vi "Process.vi"(8 "error in (no error)":errorcluster, 10 "Pound in":refnum<class "Pound.lvclass">, 11 "Qbus in":refnum<class "Qbus.lvclass">) -> (0 "error out":errorcluster)   [LabVIEW 2017, in "CmsTestPanel.lvlib"]
uses:
  <vilib>/addons/InsightCM/Devices/Shared/Cms/CmsTestPanel/CmsTestPanel.lvlib
  <vilib>/addons/Qbus/Qbus.lvclass
  <vilib>/NI/Software Watchdog/Pound/Pound.lvclass
  <vilib>/addons/InsightCM/Devices/Shared/Cms/CmsTestPanel/controls/Configuration.ctl
  <vilib>/addons/InsightCM/Devices/Shared/Common/TestPanel/controls/Configuration.ctl
  <vilib>/addons/InsightCM/Devices/Shared/Common/TestPanel/controls/State.ctl
  <vilib>/addons/InsightCM/MessageBus/Base/controls/IRoutingSource.ctl
  <vilib>/addons/TraceLogger/TraceLogger.lvlib
  <vilib>/NI/Software Watchdog/Watchdog/Watchdog.lvclass
  <vilib>/addons/InsightCM/Devices/Shared/Common/DataFlow/DataFlow.lvlib
  <vilib>/addons/InsightCM/Utilities/GlobalConfiguration/GlobalConfiguration.lvlib
  <vilib>/addons/InsightCM/Devices/Shared/Common/ServerComm/ServerComm.lvlib
  <vilib>/addons/InsightCM/Devices/Shared/Common/TestPanel/TestPanel.lvlib
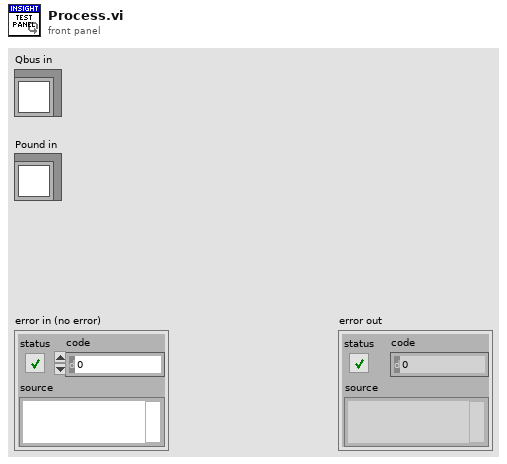
[diagram p1: front panel]
types:
  T1 = typedef "CmsTestPanel.lvlib/Configuration.ctl" = cluster{"Common":T2, "ChanNameMap":variant}
  T2 = typedef "TestPanel.lvlib/Configuration.ctl" = cluster{"State":T3, "Waveform Channel":string, "DataGroup":string, "Number of Samples":i32, "Waveform Length (sec)":dbl, "Timeout":dbl, "History":variant, "LastRequest":timestamp, "BufferSize":i32, "OpState":variant, "IRoutingSource":T4}
  T3 = typedef "TestPanel.lvlib/State.ctl" = enum16{"Off", "On", "PendingValues", "PendingDataSet"}
  T4 = typedef "IRoutingSource.ctl" = cluster{"CorrelationId":string, "ReplyTo":string}
  T5 = typedef "DataFlow.lvlib/Data.ctl" = cluster{"DataGroup":string, "Waveforms":T6, "Map":T7, "Type":T8}
  T6 = typedef "wfmSGL_DVR.ctl" = refnum<data-value>
  T7 = typedef "PointValueMap.lvlib/PointMap.ctl" = refnum<data-value>
  T8 = typedef "DataFlow.lvlib/Type.ctl" = enum16{"High Rate", "Low Rate", "Burst Mode"}
  T9 = typedef "Message.ctl" = cluster{"Header":T10, "Body":u8[]}
  T10 = typedef "MessageHeader.ctl" = cluster{"MessageName":string, "Timestamp":i64, "CorrelationId":string, "ContentType":string, "RoutingKey":string, "Properties":T11[]}
  T11 = typedef "KeyValuePair.ctl" = cluster{"Key":string, "Value":string}
  T12 = typedef "DeviceTestPanelGetTimeSeriesRequestBody.ctl" = cluster{"DataGroup":string, "TrendPointIds":string[]}
  T13 = typedef "DeviceTestPanelGetDataSetForChannelRequestBody.ctl" = cluster{"DataGroup":string, "ChannelName":string, "Properties":T11[]}
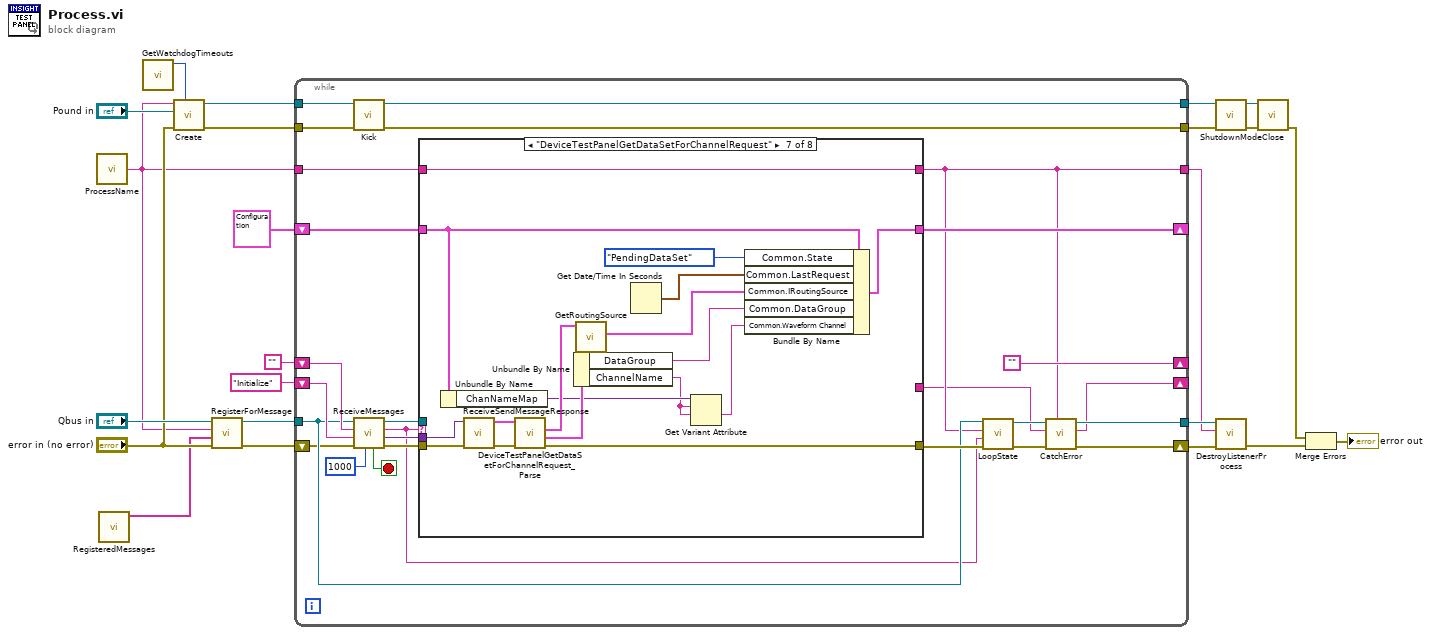
[diagram p0: block diagram]
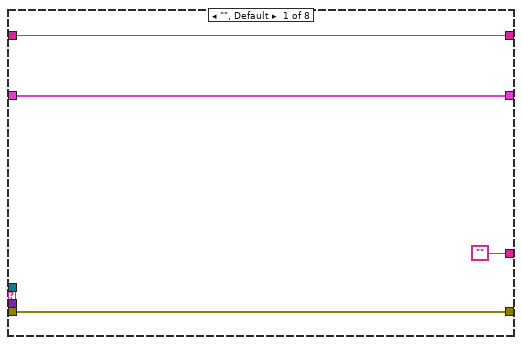
[diagram p2: hidden frame]
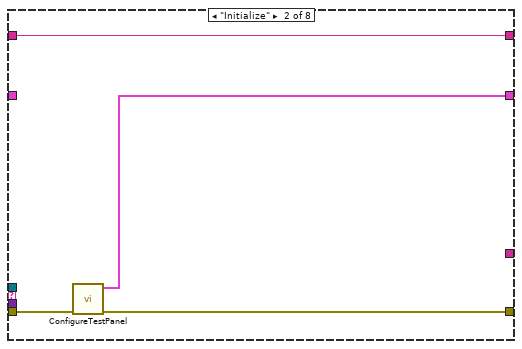
[diagram p3: hidden frame]
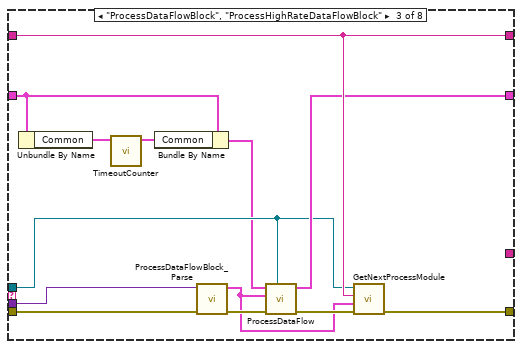
[diagram p4: hidden frame]
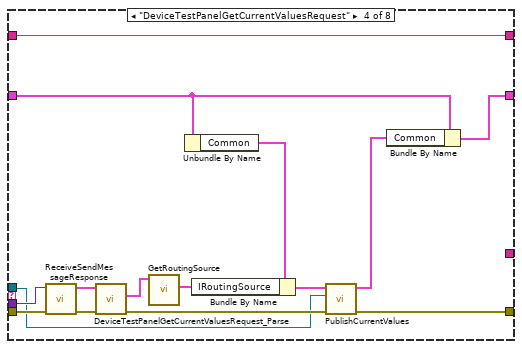
[diagram p5: hidden frame]
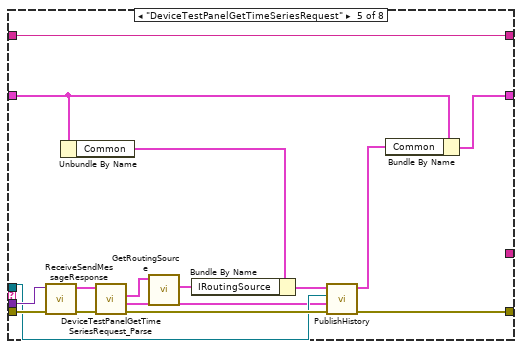
[diagram p6: hidden frame]
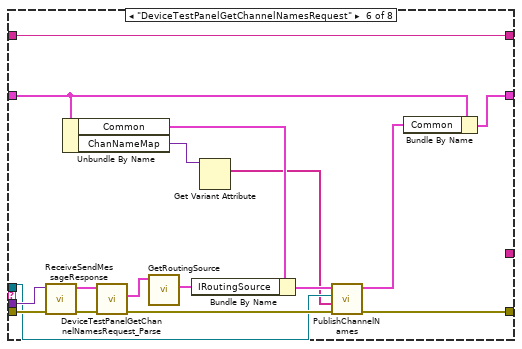
[diagram p7: hidden frame]
diagram:
  n1 = call <vilib>:"ProcessName.vi"() -> ("process name"=w3:string)  [unwired: 5 in]
  n2 = call <vilib>:"RegisteredMessages.vi"() -> ("registered messages"=w1:string[])  [unwired: 11 in]
  n3 = call <vilib>:"GetWatchdogTimeouts.vi"() -> ("software timeout"=w2:u32)  [unwired: 10 in, 1 out]
  n4 = call <vilib>:"Create.vi"("Execution Timeout (ms)"=w2, "error in (no error)"="error in (no error)", "Pound"="Pound in", "Name"=w3) -> ("error out"=w12:errorcluster, "Watchdog"=w17:refnum<data-value>)  [unwired: 6 in]
  n5 = call <vilib>:"RegisterForMessage.vi"("error in (no error)"="error in (no error)", "message names"=w1, "process name"=w3, "Qbus in"="Qbus in") -> ("error in (no error)"=w4:errorcluster, "Qbus out"=w6:refnum<class "Qbus.lvclass">)  [unwired: 6 in]
  n6 = while {
    shift-right: [""] -> _
    shift-left: "" -> [w48]
    tunnel: w6 -> [w36]
    tunnel: w3 -> [w26]
    tunnel: [w39] -> w21
    tunnel: [w25] -> w20
    shift-right: [w38] -> _
    shift-left: "Initialize" -> [w43]
    shift-right: [w41] -> _
    shift-left: T1 {"Common"={"State"=enum."Off", "Waveform Channel"="", "DataGroup"="", "Number of Samples"=0, "Waveform Length (sec)"=0.0, "Timeout"=0.0, "History"=variant, "LastRequest"=timestamp(0 s since 1904-01-01), "BufferSize"=0, "OpState"=variant, "IRoutingSource"={"CorrelationId"="", "ReplyTo"=""}}, "ChanNameMap"=variant} ("Test Panel Config") -> [w42]
    tunnel: w17 -> [w35]
    tunnel: [w34] -> w14
    tunnel: w12 -> [w33]
    tunnel: [w31] -> w11
    shift-right: [w40] -> w22
    shift-left: w4 -> [w32]
    stop <- w49 stop-if-true
    n7 = call <vilib>:"Kick.vi"("error in (no error)"=w33, "Watchdog"=w35) -> ("error out"=w31:errorcluster, "Watchdog"=w34:refnum<data-value>)  [unwired: 8 in]
    n8 = call <vilib>:"ReceiveMessages.vi"("Timeout(1000)"=1000 ("milliseconds to wait"), "error in (no error)"=w32, "priority action"=w43, "default action"=w48, "Qbus in"=w36) -> ("error out"=w47:errorcluster, "message value"=w44:variant, "action"=w30:string, "Qbus out"=w45:refnum<class "Qbus.lvclass">, "exit"=w49:bool)  [unwired: 2 in]
    n9 = case shown="\"DeviceTestPanelGetDataSetForChannelRequest\"" w30 {
      tunnel: w47 -> [w50 w57 w67 w84 w99 w116 w134 w138]
      tunnel: w45 -> [_ _ w62 w75 w87 w107 _ _]
      tunnel: [w50 w54 w69 w74 w92 w108 w128 w138] -> w37
      tunnel: w44 -> [_ _ w68 w83 w96 w115 w133 _]
      tunnel: w42 -> [w53 _ w60 w73 w89 w105 w124 w137]
      tunnel: [w53 w56 w63 w72 w88 w104 w129 w137] -> w41
      tunnel: [w52 w55 w65 w85 w101 w118 w135 w136] -> w25
      tunnel: w26 -> [w52 w55 w65 w85 w101 w118 w135 w136]
      tunnel: ["" _ _ _ _ _ _ _] -> w24
      frame "", Default {
      }
      frame "Initialize" {
        n10 = call <vilib>:"ConfigureTestPanel.vi"("error in (no error)"=w57) -> ("error out"=w54:errorcluster, "Test Panel Config out"=w56:T1)  [unwired: 9 in]
      }
      frame "ProcessDataFlowBlock", "ProcessHighRateDataFlowBlock" {
        n11 = Unbundle By Name(w60) -> ("Common"=w61:T2)
        n12 = call <vilib>:"TimeoutCounter.vi"("config in"=w61) -> ("config out"=w59:T2)  [unwired: 10 in]
        n13 = Bundle By Name(cluster=w60, "Common"=w59) -> (w58:T1)
        n14 = call <vilib>:"ProcessDataFlowBlock_Parse.vi"("error in (no error)"=w67, "body"=w68) -> ("error out"=w66:errorcluster, "data"=w64:T5)  [unwired: 8 in]
        n15 = call <vilib>:"ProcessDataFlow.vi"("Qbus in"=w62, "error in (no error)"=w66, "Data"=w64, "config in"=w58) -> ("error out"=w70:errorcluster, "config out"=w63:T1)  [unwired: 6 in]
        n16 = call <vilib>:"GetNextProcessModule.vi"("error in (no error)"=w70, "data"=w64, "source"=w65, "Qbus in"=w62) -> ("error out"=w69:errorcluster)  [unwired: 6 in, 1 out]
      }
      frame "DeviceTestPanelGetCurrentValuesRequest" {
        n17 = call <vilib>:"ReceiveSendMessageResponse.vi"("error in (no error)"=w84, "body"=w83) -> ("error out"=w82:errorcluster, "message"=w81:T9)  [unwired: 6 in, 2 out]
        n18 = call <vilib>:"DeviceTestPanelGetCurrentValuesRequest_Parse.vi"("error in (no error)"=w82, "Message"=w81) -> ("error out"=w76:errorcluster, "Header"=w80:T10)  [unwired: 7 in, 1 out]
        n19 = call <vilib>:"GetRoutingSource.vi"("Header in"=w80) -> ("IRoutingSource"=w79:T4)  [unwired: 9 in, 1 out]
        n20 = Unbundle By Name(w73) -> ("Common"=w78:T2)
        n21 = Bundle By Name(cluster=w78, "IRoutingSource"=w79) -> (w77:T2)
        n22 = call <vilib>:"PublishCurrentValues.vi"("error in (no error)"=w76, "Qbus in"=w75, "config in"=w77) -> ("error out"=w74:errorcluster, "config out"=w71:T2)  [unwired: 7 in]
        n23 = Bundle By Name(cluster=w73, "Common"=w71) -> (w72:T1)
      }
      frame "DeviceTestPanelGetTimeSeriesRequest" {
        n24 = call <vilib>:"ReceiveSendMessageResponse.vi"("error in (no error)"=w99, "body"=w96) -> ("error out"=w98:errorcluster, "message"=w97:T9)  [unwired: 6 in, 2 out]
        n25 = Unbundle By Name(w89) -> ("Common"=w94:T2)
        n26 = call <vilib>:"DeviceTestPanelGetTimeSeriesRequest_Parse.vi"("error in (no error)"=w98, "Message"=w97) -> ("error out"=w93:errorcluster, "Body"=w86:T12, "Header"=w95:T10)  [unwired: 6 in, 1 out]
        n27 = call <vilib>:"GetRoutingSource.vi"("Header in"=w95) -> ("IRoutingSource"=w100:T4)  [unwired: 9 in, 1 out]
        n28 = Bundle By Name(cluster=w94, "IRoutingSource"=w100) -> (w91:T2)
        n29 = call <vilib>:"PublishHistory.vi"("error in (no error)"=w93, "Body"=w86, "Qbus in"=w87, "config in"=w91) -> ("error out"=w92:errorcluster, "config out"=w90:T2)  [unwired: 6 in]
        n30 = Bundle By Name(cluster=w89, "Common"=w90) -> (w88:T1)
      }
      frame "DeviceTestPanelGetChannelNamesRequest" {
        n31 = call <vilib>:"ReceiveSendMessageResponse.vi"("error in (no error)"=w116, "body"=w115) -> ("error out"=w113:errorcluster, "message"=w114:T9)  [unwired: 6 in, 2 out]
        n32 = Unbundle By Name(w105) -> ("Common"=w111:T2, "ChanNameMap"=w103:variant)
        n33 = call <vilib>:"DeviceTestPanelGetChannelNamesRequest_Parse.vi"("error in (no error)"=w113, "Message"=w114) -> ("error out"=w109:errorcluster, "Header"=w112:T10)  [unwired: 7 in, 1 out]
        n34 = call <vilib>:"GetRoutingSource.vi"("Header in"=w112) -> ("IRoutingSource"=w117:T4)  [unwired: 9 in, 1 out]
        n35 = Bundle By Name(cluster=w111, "IRoutingSource"=w117) -> (w110:T2)
        n36 = Get Variant Attribute(Variant=w103) -> (names=w102:string[])  [unwired: 3 in, 3 out]
        n37 = call <vilib>:"PublishChannelNames.vi"("error in (no error)"=w109, "names"=w102, "Qbus in"=w107, "config in"=w110) -> ("error out"=w108:errorcluster, "config out"=w106:T2)  [unwired: 6 in]
        n38 = Bundle By Name(cluster=w105, "Common"=w106) -> (w104:T1)
      }
      frame "DeviceTestPanelGetDataSetForChannelRequest" {
        n39 = Unbundle By Name(w124) -> ("ChanNameMap"=w123:variant)
        n40 = call <vilib>:"ReceiveSendMessageResponse.vi"("error in (no error)"=w134, "body"=w133) -> ("error out"=w131:errorcluster, "message"=w132:T9)  [unwired: 6 in, 2 out]
        n41 = call <vilib>:"DeviceTestPanelGetDataSetForChannelRequest_Parse.vi"("error in (no error)"=w131, "Message"=w132) -> ("error out"=w128:errorcluster, "Body"=w130:T13, "Header"=w126:T10)  [unwired: 6 in, 1 out]
        n42 = Unbundle By Name(w130) -> ("DataGroup"=w121:string, "ChannelName"=w122:string)
        n43 = call <vilib>:"GetRoutingSource.vi"("Header in"=w126) -> ("IRoutingSource"=w125:T4)  [unwired: 9 in, 1 out]
        n44 = Get Date/Time In Seconds() -> (seconds since 1Jan1904=w127:timestamp)
        n45 = Get Variant Attribute(Variant=w123, name=w122, default value (empty Variant)=w122) -> (value=w120:string)  [unwired: 1 in, 3 out]
        n46 = Bundle By Name(cluster=w124, "Common.State"=State."PendingDataSet" ("Test Panel State"), "Common.LastRequest"=w127, "Common.IRoutingSource"=w125, "Common.DataGroup"=w121, "Common.Waveform Channel"=w120) -> (w129:T1)
      }
      frame "Exit" {
      }
    }
    n47 = call <vilib>:"LoopState.vi"("error in (no error)"=w37, "loop action"=w30, "process name"=w25, "Qbus in"=w36) -> ("error out"=w28:errorcluster, "Qbus out"=w27:refnum<class "Qbus.lvclass">)  [unwired: 6 in]
    n48 = call <vilib>:"CatchError.vi"("source"=w25, "error in (no error)"=w28, "next action in"=w24, "Qbus in"=w27) -> ("error out"=w40:errorcluster, "next action out"=w38:string, "Qbus out"=w39:refnum<class "Qbus.lvclass">)  [unwired: 5 in]
  }
  n49 = call <vilib>:"ShutdownMode.vi"("error in (no error)"=w11, "Watchdog"=w14) -> ("error out"=w13:errorcluster, "Watchdog"=w15:refnum<data-value>)  [unwired: 8 in]
  n50 = call <vilib>:"DestroyListenerProcess.vi"("error in (no error)"=w22, "process name"=w20, "Qbus in"=w21) -> ("error in (no error)"=w10:errorcluster)  [unwired: 7 in, 1 out]
  n51 = call <vilib>:"Close.vi"("error in (no error)"=w13, "Watchdog"=w15) -> ("error out"=w9:errorcluster)  [unwired: 9 in]
  n52 = Merge Errors(w9, w10) -> (→"error out":errorcluster)
